vi "Calibrate Theta.vi"(8 "error constant":errorcluster, 11 "Modules":refnum<class "Module.lvclass">[](array[class])) -> (3 "Continue?":bool)   [LabVIEW 2021, in "Module.lvclass"]
uses:
  Module.lvclass
  Module.lvclass/Module.ctl
panel:
  in  "Again":bool
  in  "Move On":bool
  out "Theta":cluster{i32[], dbl[]}[](graph)
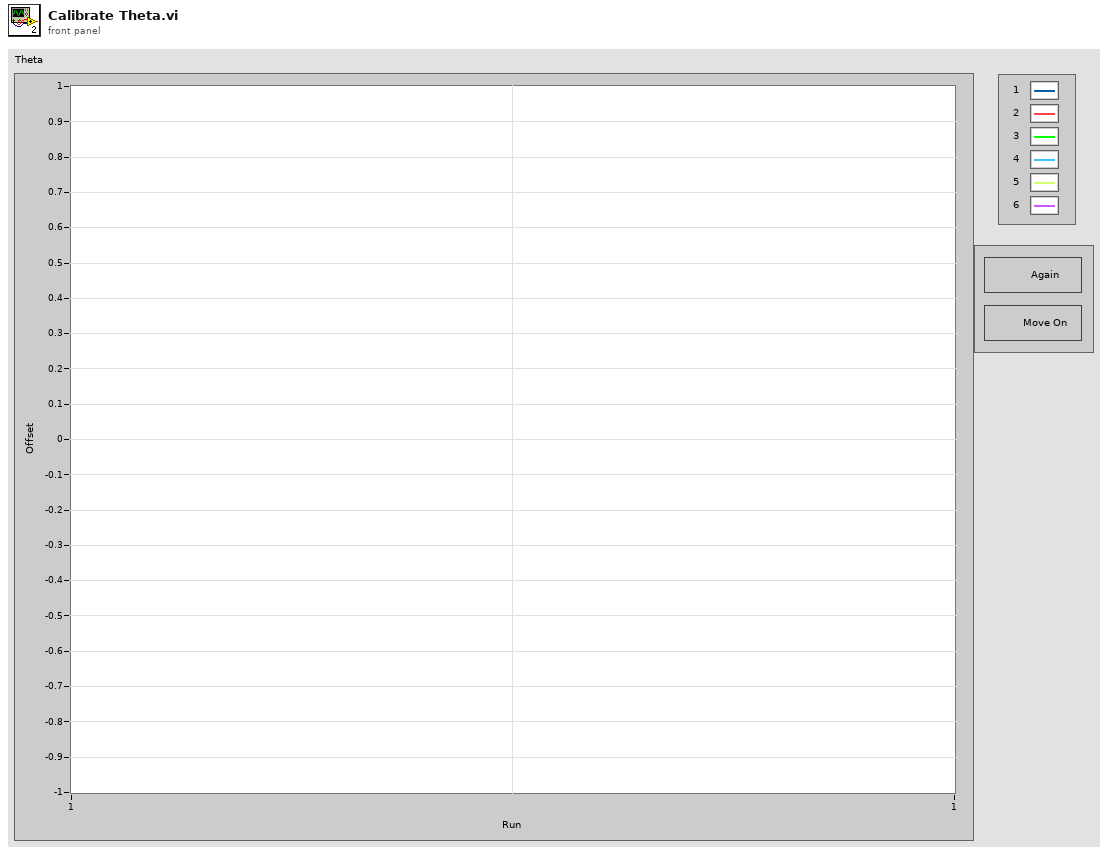
[diagram p1: front panel]
types:
  T1 = typedef "File Paths.ctl" = cluster{"Glue Pattern Folder":path, "Carrier Tray Folder":path, "Pick Up Tool Fixture Folder":path, "Components Folder":path, "Bellows Tool Offset.txt":path, "Pick Up Tool Offset.txt":path, "Dispense Tip Offset.txt":path, "Log Files":path, "Gantry Assembly Map.txt":path, "Syringe and offset map.txt":path, "Python DB Conn":path}
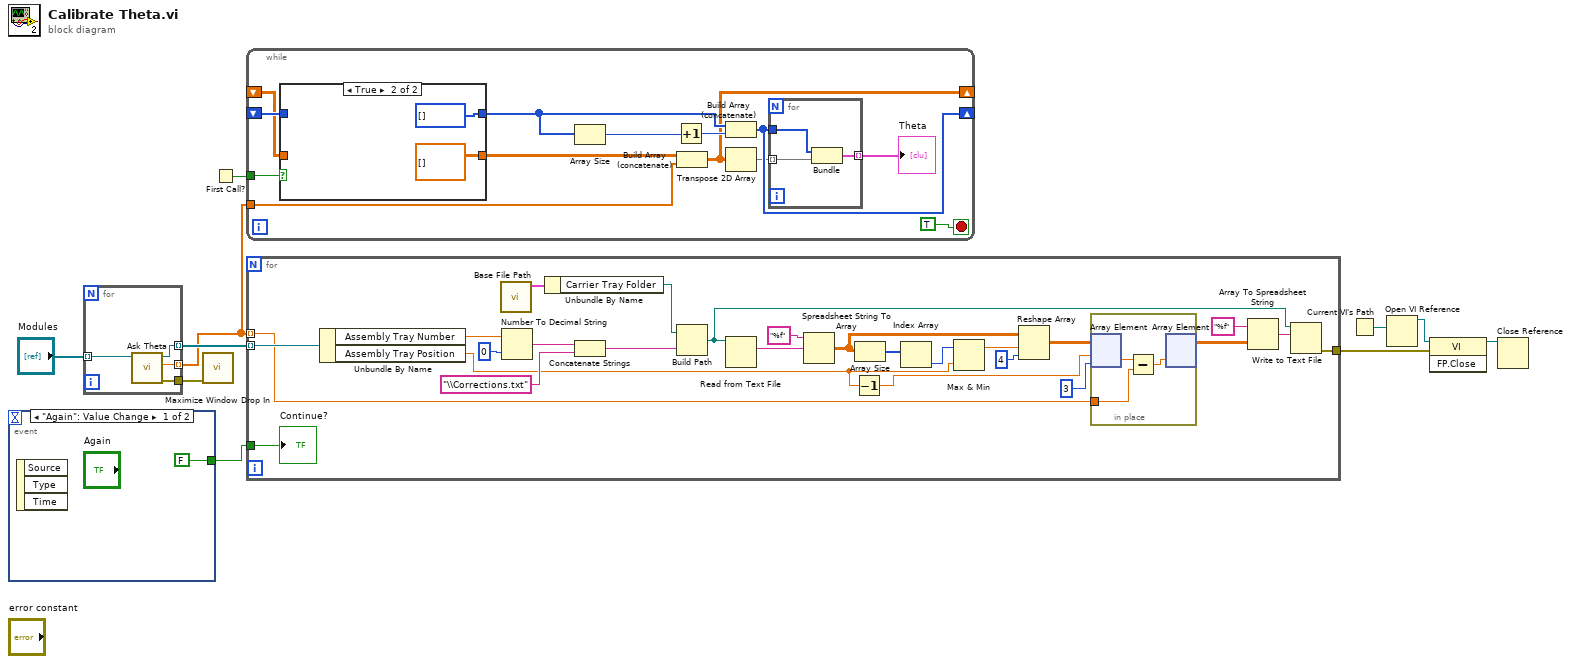
[diagram p0: block diagram]
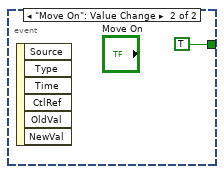
[diagram p3: hidden frame]
diagram:
  n1 = event shown="[0] \"Again\": Value Change" {
    selector: _ -> [_ _]
    dyn-events: _ -> [_ _]
    timeout: _ -> [_ _]
    tunnel: [FALSE TRUE] -> w10
    event "Again": Value Change {
      n2 = event-data() -> ()  [unwired: 1 in, 3 out]
    }
    event "Move On": Value Change {
      n3 = event-data() -> ()  [unwired: 1 in, 6 out]
    }
  }
  n4 = for {
    tunnel: "Modules" -> [w16] mode=indexing
    tunnel: [w15] -> w7 mode=indexing
    tunnel: [w14] -> w6 mode=indexing
    tunnel: [w13] -> w2
    n5 = call "Ask Theta.vi"("Module in"=w16) -> ("error out"=w13:errorcluster, "Theta Error Out"=w14:dbl, "Module out"=w15:refnum<class "Module.lvclass">)  [unwired: 8 in]
  }
  n6 = call "Maximize Window Drop In.vi"("error out 2"=w2) -> ()  [unwired: 10 in, 1 out]
  n7 = First Call?() -> (First Call?: T/F=w8:bool)
  n8 = while {
    tunnel: w6 -> [w28]
    tunnel: w8 -> [w29]
    shift-right: [w19] -> _
    shift-left: _ -> [w24]
    shift-right: [w20] -> _
    shift-left: _ -> [w27]
    stop <- TRUE stop-if-true
    n9 = case shown="True" w29 {
      tunnel: [w33 i32[] []] -> w21
      tunnel: w27 -> [w33 _]
      tunnel: [w34 dbl[][] []] -> w25
      tunnel: w24 -> [w34 _]
      frame False {
      }
      frame True {
      }
    }
    n10 = Array Size(array=w21) -> (size(s)=w22:i32)
    n11 = Increment(x=w22) -> (x+1=w23:i32)
    n12 = Build Array (concatenate)(w25, w28) -> (w19:dbl[][])
    n13 = Build Array (concatenate)(w21, w23) -> (w20:i32[])
    n14 = Transpose 2D Array(2D array=w19) -> (transposed array=w18:dbl[][])
    n15 = for {
      tunnel: w18 -> [w30] mode=indexing
      tunnel: [w32] -> w17 mode=indexing
      tunnel: w20 -> [w31]
      n16 = Bundle(w31, w30) -> (w32:cluster{i32[], dbl[]})  [unwired: 1 in]
    }
    "Theta" <- w17
  }
  n17 = for {
    tunnel: w10 -> [w62]
    tunnel: w7 -> [w47] mode=indexing
    tunnel: w6 -> [w45] mode=indexing
    tunnel: [w44] -> w4
    n18 = Unbundle By Name(w47) -> ("Assembly Tray Number"=w46:dbl, "Assembly Tray Position"=w38:dbl)
    n19 = call "Base File Path.vi"() -> ("Paths Out"=w61:T1)  [unwired: 11 in]
    n20 = Number To Decimal String(number=w46, width (-)=i16 0) -> (decimal integer string=w58:string)
    n21 = Unbundle By Name(w61) -> ("Carrier Tray Folder"=w60:path)
    n22 = Concatenate Strings(w58, "\\Corrections.txt" ("string")) -> (w56:string)
    n23 = Build Path(base path=w60, name or relative path=w56) -> (appended path=w53:path)
    n24 = Read from Text File(file (use dialog)=w53) -> (text=w55:string)  [unwired: 3 in, 3 out]
    n25 = Spreadsheet String To Array(format string="%f", spreadsheet string=w55) -> (array=w40:dbl[][])  [unwired: 2 in]
    n26 = Decrement(x=w38) -> (x-1=w52:dbl)
    n27 = Array Size(array=w40) -> (size(s)=w42:i32[])
    n28 = Index Array(array=w42) -> (element=w39:i32)  [unwired: 1 in]
    n29 = Max & Min(x=w39, y=w38) -> (max(x,y)=w43:dbl)  [unwired: 1 out]
    n30 = Reshape Array(w40, w43, 4 ("dimension size")) -> (w37:dbl[][])
    n31 = in-place {
      in-place-border: w45 -> [w64]
      n32 = in-place-array #1(w37, w52, 3 ("disabled index (col)")) -> (w65:dbl)
      n33 = Subtract(x=w65, y=w64) -> (x-y=w63:dbl)
      n34 = in-place-array #1(w63) -> (w50:dbl[][])  [unwired: 2 out]
    }
    n35 = Array To Spreadsheet String(array=w50, 3:"%f" ("format string")) -> (spreadsheet string=w48:string)  [unwired: 1 in]
    n36 = Write to Text File(file (use dialog)=w53, text=w48) -> (error out=w44:errorcluster)  [unwired: 2 in, 2 out]
    "Continue?" <- w62
  }
  n37 = Current VI's Path() -> (path=w5:path)
  n38 = Open VI Reference(vi path=w5) -> (vi reference=w1:refnum<vi>)  [unwired: 5 in, 1 out]
  n39 = invoke class="VI" method="FP.Close"(reference=w1, error in=w4) -> (reference out=w3:refnum<vi>)  [unwired: 1 in, 2 out]
  n40 = Close Reference(reference=w3) -> ()  [unwired: 1 in, 1 out]
